vi "Undo.vi"(0 "User Manager View in":refnum<class "User Manager View.lvclass">, 11 "error in (no error)":errorcluster) -> (4 "User Manager View out":refnum<class "User Manager View.lvclass">, 15 "error out":errorcluster)   [LabVIEW 2017, in "User Manager View.lvlib" / "User Manager View.lvclass"]
uses:
  <vilib>/gpm_packages/@cs/User Manager App/User Manager View/User Manager View/User Manager View.lvclass
  C:/Program Files/National Instruments/LabVIEW 2017/vi.lib/ActorFramework/Actor/Actor.lvclass
  <vilib>/gpm_packages/@cs/User Manager App/User Manager View/User Manager Type Defs/State.ctl
  <vilib>/ActorFramework/Actor/Actor.lvclass/Actor.ctl
  <vilib>/ActorFramework/Message Enqueuer/Message Enqueuer.lvclass/Message Enqueuer.ctl
  <vilib>/gpm_packages/@cs/User Manager App/User Manager View/User Manager View/User Manager View.lvclass/User Manager View.ctl
  <vilib>/gpm_packages/@cs/User Manager App/User Manager View/User Manager View Messages/Pick User Msg/Pick User Msg.lvclass/Pick User Msg.ctl
  <vilib>/ActorFramework/Message Enqueuer/Init from Existing Queue.vi
  <vilib>/ActorFramework/Message Enqueuer/Enqueue.vi
  <vilib>/gpm_packages/@cs/User Manager App/User Manager View/User Manager View Messages/Pick User Msg/Pick User Msg.lvclass
  C:/Program Files/National Instruments/LabVIEW 2017/vi.lib/ActorFramework/Message/Message.lvclass
  <vilib>/ActorFramework/Message Priority Queue/Priority Enqueue.vi
  <vilib>/ActorFramework/Message Enqueuer/Message Enqueuer.lvclass
  <vilib>/gpm_packages/@cs/User Manager App/User Manager View/User Manager View.lvlib
  <vilib>/ActorFramework/Actor/Actor.lvclass
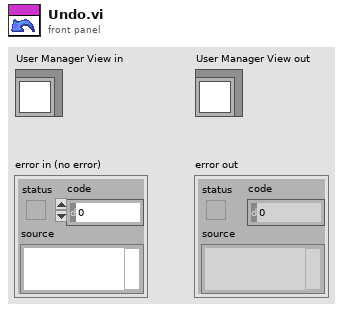
[diagram p1: front panel]
types:
  T1 = enum8{"Enabled", "Disabled", "Disabled and Grayed Out"}
  T2 = typedef "User Manager View.lvlib/State.ctl" = enum16{"Normal", "Adding User", "Changing User Data"}
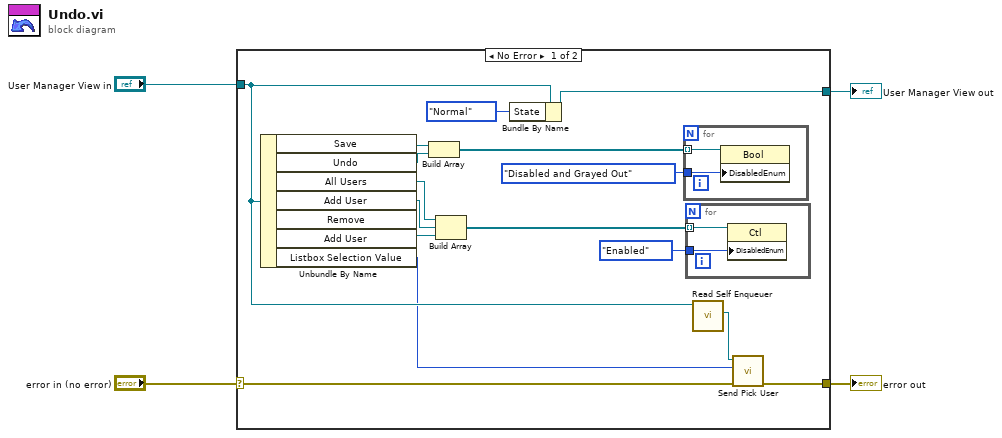
[diagram p0: block diagram]
diagram:
  n1 = case shown="No Error" "error in (no error)" {
    selector: "error in (no error)" -> [w6 w26]
    tunnel: [w5 w26] -> w3
    tunnel: [w19 w25] -> w1
    tunnel: "User Manager View in" -> [w18 w25]
    frame No Error {
      n2 = Unbundle By Name(w18) -> ("Save"=w9:refnum<vi>, "Undo"=w10:refnum<vi>, "All Users"=w15:refnum<vi>, "Add User"=w14:refnum<vi>, "Remove"=w8:refnum<vi>, "Listbox Selection Value"=w7:i32)  [unwired: 1 out]
      n3 = Build Array(w9, w10) -> (w12:refnum<vi>[])
      n4 = Build Array(w15, w14, w8) -> (w13:refnum<vi>[])
      n5 = Bundle By Name(cluster=w18, "State"=State."Normal") -> (w19:refnum<class "User Manager View.lvclass">)
      n6 = for {
        tunnel: w12 -> [w22] mode=indexing
        tunnel: T1."Disabled and Grayed Out" ("Disabled") -> [w21]
        n7 = property class="Bool"(reference=w22, "DisabledEnum"=w21) -> ()  [unwired: 1 in, 2 out]
      }
      n8 = for {
        tunnel: w13 -> [w24] mode=indexing
        tunnel: T1."Enabled" ("Disabled") -> [w23]
        n9 = property class="Ctl"(reference=w24, "DisabledEnum"=w23) -> ()  [unwired: 1 in, 2 out]
      }
      n10 = call <vilib>:"Read Self Enqueuer.vi"("Actor"=w18) -> ("Self Enqueuer"=w17:refnum<class "Message Enqueuer.lvclass">)  [unwired: 10 in]
      n11 = call <vilib>:"Send Pick User.vi"("error in (no error)"=w6, "NewVal"=w7, "Message Enqueuer"=w17) -> ("error out"=w5:errorcluster)  [unwired: 7 in, 1 out]
    }
    frame Error {
    }
  }
  "error out" <- w3
  "User Manager View out" <- w1
